vi "Client Init Test.vi"() -> (0 "no error":errorcluster, 1 "tags found":bool, 2 "expected execution settings":bool)   [LabVIEW 2014, in "OPC UA Client Tests.lvlib"]
doc: "Tests Init override for client configuration"
uses:
  OPC UA Client Tests.lvlib
  module/execution/OPC UA Client runtime.lvclass
  Server Connection Configuration.ctl
  <vilib>/OPCUA/server/subVI/supported security policies.ctl
  module/configuration/Client Connection Configuration.ctl
  module/configuration/OPC UA Client configuration.lvclass/OPC UA Client configuration.ctl
  <vilib>/NI/Tag Bus/tag/tag descriptor.lvclass/tag descriptor.ctl
  <vilib>/NI/Tag Bus Module Framework/channel/TBM channel.lvclass/TBM channel.ctl
  <vilib>/NI/Tag Bus/tag/read tag name.vi
  <vilib>/NI/Tag Bus/tag/read data type.vi
  <vilib>/NI/Tag Bus Module Framework/channel/Read channel classification.vi
  module/configuration/Read Lines.vi
  <vilib>/NI/Tag Bus Module Framework/channel/TBM channel.lvclass
  module/configuration/OPC UA Client configuration.lvclass
  <vilib>/NI/Tag Bus/dictionary/data dictionary.lvclass
  <vilib>/opcua/NI OPC UA Server.lvlib
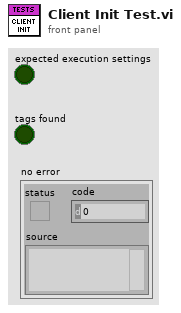
[diagram p1: front panel]
types:
  T1 = typedef "OPC UA Client configuration.lvclass/Client Connection Configuration.ctl" = cluster{"Server Certificates":cluster{"Relative Path?":bool, "Server Paths":string[]}, "Client Certificates":cluster{"Relative Path?":bool, "Client Path":string}, "Client Configuration":cluster{"Server Endpoint URL":string, "Security Policy":cluster{"Message Mode":enum16{"None", "Sign", "Sign and Encrypt"}, "Security":enum16{"Basic256", "Basic128Rsa15"}}, "Username/Password":cluster{"Username":string, "Password":string}}}
  T2 = typedef "OPC UA Client Tests.lvlib/Server Connection Configuration.ctl" = cluster{"Server Certificates":cluster{"Relative Path?":bool, "Certificate Paths":path[], "Certificate Names":string[]}, "Client Certificates":cluster{"Relative Path?":bool, "Certificate Paths":path[], "Certificate Names":string[]}, "Server Configuration":cluster{"Server Name":string, "TCP port (49580)":string, "Supported Security Policies":T3}}
  T3 = typedef "supported security policies.ctl" = cluster{"None":bool, "Sign with Basic128Rsa125":bool, "Sign and Encrypt with Basic128Rsa125":bool, "Sign with Basic256":bool, "Sign and Encrypt with Basic256":bool}
  T4 = typedef "OPC UA configuration.lvclass/Line.ctl" = cluster{"channel":refnum<class "TBM channel.lvclass">, "Node Path":string, "OPC UA Data Type":T5}
  T5 = typedef "OPC UA configuration.lvclass/OPC UA Data Type.ctl" = u16
  T6 = typedef "TBM channel.lvclass/data tables.ctl" = cluster{"input data":T7, "processing parameter":T7, "processing result":T7, "output data":T7}
  T7 = typedef "tag bus.lvlib/dictionary table pair.ctl" = cluster{"data dictionary":refnum<class "data dictionary.lvclass">, "data table":T8}
  T8 = typedef "tag bus.lvlib/data table.lvlib/data table.ctl" = cluster{"Double":dbl[], "Single":sgl[], "I64":i64[], "I32":i32[], "I16":i16[], "I8":i8[], "U64":u64[], "U32":u32[], "U16":u16[], "U8":u8[], "Boolean":bool[], "String":string[], "Array of Double":cluster{"DBL Array":dbl[]}[], "Array of Single":cluster{"SGL Array":sgl[]}[], "Array of I64":cluster{"I64 Array":i64[]}[], "Array of I32":cluster{"I32 Array":i32[]}[], "Array of I16":cluster{"I16 Array":i16[]}[], "Array of I8":cluster{"I8 Array":i8[]}[], "Array of U64":cluster{"U64 Array":u64[]}[], "Array of U32":cluster{"U32 Array":u32[]}[], "Array of U16":cluster{"U16 Array":u16[]}[], "Array of U8":cluster{"U8 Array":u8[]}[], "Array of Boolean":cluster{"Boolean Array":bool[]}[], "Array of String":cluster{"String Array":string[]}[]}
  T9 = typedef "TBM module execution interface.lvclass/execution settings.ctl" = cluster{"reads inputs":bool, "processes data":bool, "writes outputs":bool}
  T10 = typedef "tag bus.lvlib/tag descriptor.lvclass/Data Type.ctl" = enum16{"Double", "Single", "I64", "I32", "I16", "I8", "U64", "U32", "U16", "U8", "Boolean", "String", "Array of Double", "Array of Single", "Array of I64", "Array of I32", "Array of I16", "Array of I8", "Array of U64", "Array of U32", "Array of U16", "Array of U8", "Array of Boolean", "Array of String"}
  T11 = typedef "TBM channel.lvclass/channel classification.ctl" = enum16{"input data", "output data", "processing parameter", "processing result"}
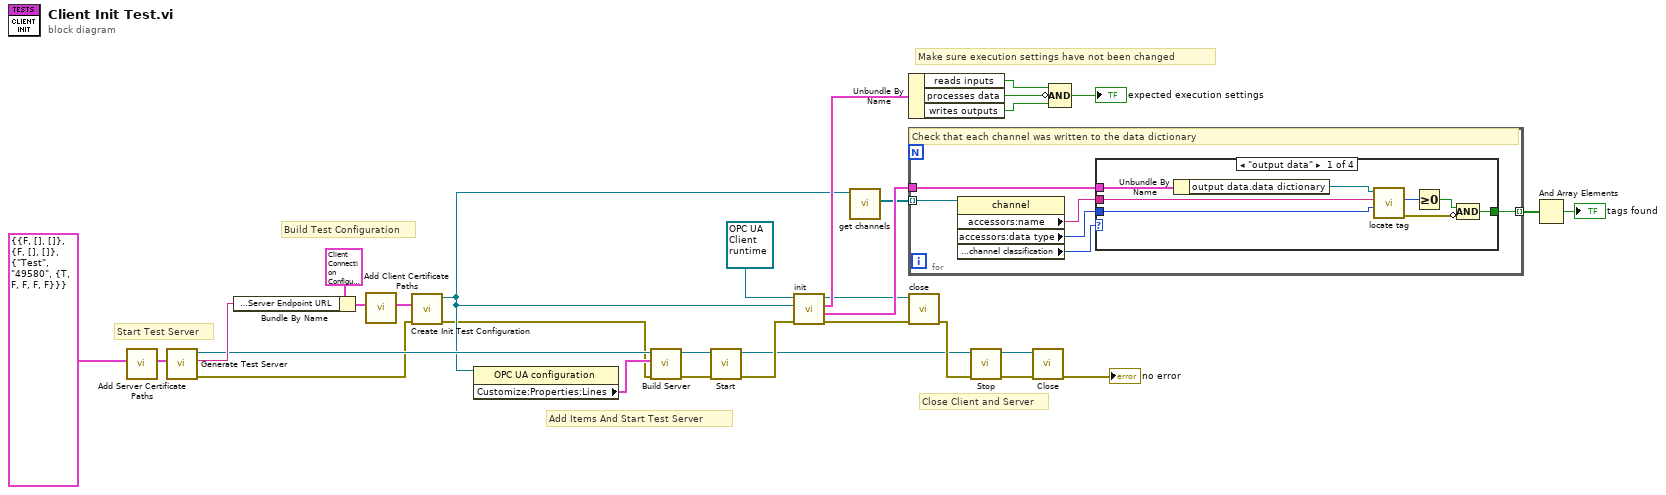
[diagram p0: block diagram]
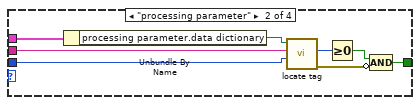
[diagram p2: hidden frame]
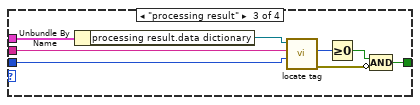
[diagram p3: hidden frame]
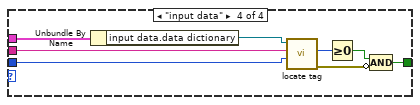
[diagram p4: hidden frame]
diagram:
  # "Make sure execution settings have not been changed"
  # "Close Client and Server"
  # "Add Items And Start Test Server"
  # "Start Test Server"
  # "Build Test Configuration"
  n1 = call "Add Server Certificate Paths.vi"("Server Connection Configuration In"=T2 {"Server Certificates"={"Relative Path?"=FALSE, "Certificate Paths"=[], "Certificate Names"=[]}, "Client Certificates"={"Relative Path?"=FALSE, "Certificate Paths"=[], "Certificate Names"=[]}, "Server Configuration"={"Server Name"="Test", "TCP port (49580)"="49580", "Supported Security Policies"={"None"=TRUE, "Sign with Basic128Rsa125"=FALSE, "Sign and Encrypt with Basic128Rsa125"=FALSE, "Sign with Basic256"=FALSE, "Sign and Encrypt with Basic256"=FALSE}}}) -> ("Server Connection Configuration Out"=w8:T2)  [unwired: 10 in]
  n2 = call "Generate Test Server.vi"("Server Connection Configuration"=w8) -> ("OPC UA server refnum out"=w19:refnum<k21>, "server endpoint URL"=w20:string, "error out"=w4:errorcluster)  [unwired: 7 in]
  n3 = Bundle By Name(cluster=T1 {"Server Certificates"={"Relative Path?"=FALSE, "Server Paths"=[]}, "Client Certificates"={"Relative Path?"=FALSE, "Client Path"=""}, "Client Configuration"={"Server Endpoint URL"="", "Security Policy"={"Message Mode"=enum."None", "Security"=enum."Basic256"}, "Username/Password"={"Username"="", "Password"=""}}} ("Client Connection Configuration"), "Client Configuration.Server Endpoint URL"=w20) -> (w6:T1)
  n4 = call "Add Client Certificate Paths.vi"("Client Connection Configuration In"=w6) -> ("Client Connection Configuration Out"=w5:T1)  [unwired: 10 in]
  n5 = call "Create Init Test Configuration.vi"("error in"=w4, "Connection Configuration"=w5) -> ("error out"=w16:errorcluster, "module"=w18:refnum<class "OPC UA Client configuration.lvclass">)  [unwired: 7 in, 1 out]
  n6 = property class="OPC UA configuration"(reference=w18) -> ("Customize:Properties:Lines"=w17:T4[])  [unwired: 1 in, 2 out]
  n7 = call "Build Server.vi"("Error In"=w16, "Lines"=w17, "OPC UA server refnum in"=w19) -> ("Error Out"=w15:errorcluster, "OPC UA server refnum out"=w12:refnum<k21>)  [unwired: 7 in]
  n8 = call <vilib>:"Start.vi"("error in (no error)"=w15, "OPC UA server refnum in"=w12) -> ("error out"=w13:errorcluster, "OPC UA server refnum out"=w11:refnum<k21>)  [unwired: 8 in]
  n9 = call-dynamic "init.vi"("error in"=w13, "TBM module configuration in"=w18, "OPC UA runtime in"=refnum<class "OPC UA Client runtime.lvclass"> refnum ("OPC UA runtime")) -> ("error out"=w23:errorcluster, "data allocations"=w31:T6, "execution settings"=w30:T9, "OPC UA runtime out"=w21:refnum<class "OPC UA Client runtime.lvclass">)  [unwired: 5 in]
  n10 = call-dynamic "get channels.vi"("OPC UA configuration in"=w18) -> ("channels"=w22:refnum<class "TBM channel.lvclass">[])  [unwired: 9 in, 1 out]
  n11 = Unbundle By Name(w30) -> ("reads inputs"=w29:bool, "processes data"=w27:bool, "writes outputs"=w28:bool)
  n12 = for {
    tunnel: w31 -> [w37]
    tunnel: w22 -> [w36] mode=indexing
    tunnel: [w35] -> w25 mode=indexing
    # "Check that each channel was written to the data dictionary"
    n13 = property class="channel"(reference=w36) -> ("accessors:name"=w32:string, "accessors:data type"=w33:T10, "data access:channel classification"=w34:T11)  [unwired: 1 in, 2 out]
    n14 = case shown="\"output data\"" w34 {
      tunnel: w37 -> [w45 w53 w61 w69]
      tunnel: w33 -> [w43 w51 w59 w67]
      tunnel: w32 -> [w42 w50 w58 w66]
      tunnel: [w38 w46 w54 w62] -> w35
      frame "output data" {
        n15 = Unbundle By Name(w45) -> ("output data.data dictionary"=w44:refnum<class "data dictionary.lvclass">)
        n16 = call <vilib>:"locate tag.vi"("data type"=w43, "name"=w42, "data dictionary in"=w44) -> ("error out"=w39:errorcluster, "index"=w41:i32)  [unwired: 6 in, 1 out]
        n17 = Greater Or Equal To 0?(x=w41) -> (x >= 0?=w40:bool)
        n18 = Compound Arithmetic op=AND(w40, invert w39) -> (w38:bool)
      }
      frame "processing parameter" {
        n19 = Unbundle By Name(w53) -> ("processing parameter.data dictionary"=w52:refnum<class "data dictionary.lvclass">)
        n20 = call <vilib>:"locate tag.vi"("data type"=w51, "name"=w50, "data dictionary in"=w52) -> ("error out"=w47:errorcluster, "index"=w49:i32)  [unwired: 6 in, 1 out]
        n21 = Greater Or Equal To 0?(x=w49) -> (x >= 0?=w48:bool)
        n22 = Compound Arithmetic op=AND(w48, invert w47) -> (w46:bool)
      }
      frame "processing result" {
        n23 = Unbundle By Name(w61) -> ("processing result.data dictionary"=w60:refnum<class "data dictionary.lvclass">)
        n24 = call <vilib>:"locate tag.vi"("data type"=w59, "name"=w58, "data dictionary in"=w60) -> ("error out"=w55:errorcluster, "index"=w57:i32)  [unwired: 6 in, 1 out]
        n25 = Greater Or Equal To 0?(x=w57) -> (x >= 0?=w56:bool)
        n26 = Compound Arithmetic op=AND(w56, invert w55) -> (w54:bool)
      }
      frame "input data" {
        n27 = Unbundle By Name(w69) -> ("input data.data dictionary"=w68:refnum<class "data dictionary.lvclass">)
        n28 = call <vilib>:"locate tag.vi"("data type"=w67, "name"=w66, "data dictionary in"=w68) -> ("error out"=w63:errorcluster, "index"=w65:i32)  [unwired: 6 in, 1 out]
        n29 = Greater Or Equal To 0?(x=w65) -> (x >= 0?=w64:bool)
        n30 = Compound Arithmetic op=AND(w64, invert w63) -> (w62:bool)
      }
    }
  }
  n31 = call-dynamic <vilib>:"close.vi"("error in"=w23, "OPC UA runtime in"=w21) -> ("error out"=w14:errorcluster)  [unwired: 9 in]
  n32 = call <vilib>:"Stop.vi"("error in (no error)"=w14, "OPC UA server refnum in"=w11) -> ("error out"=w3:errorcluster, "OPC UA server refnum out"=w2:refnum<k21>)  [unwired: 8 in]
  n33 = call <vilib>:"Close.vi"("error in (no error)"=w3, "OPC UA server refnum in"=w2) -> ("error out"=→"no error":errorcluster)  [unwired: 9 in]
  n34 = Compound Arithmetic op=AND(w29, invert w27, w28) -> (→"expected execution settings":bool)
  n35 = And Array Elements(Boolean array=w25) -> (logical AND=→"tags found":bool)
